vi "Get Drive List.vi"(7 "error in (no error)":errorcluster) -> (0 "error out":errorcluster, 3 "驱动器列表":string[](array[string]))   [LabVIEW 2012, in "API.lvlib"]
doc: "Uses an API call to retrieve a list of all available drives.\nThe output is an array of strings (one element for each drive letter)\nof the format \"c:\\\""
uses:
  API.lvlib
  kernel32.dll
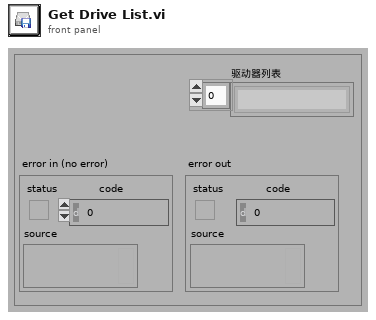
[diagram p1: front panel]
types:
  T1 = enum16{"big-endian, network order", "native, host order", "little-endian"}
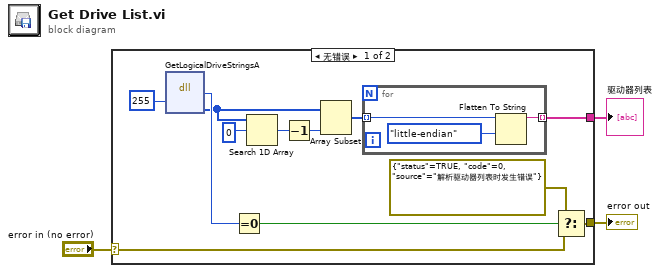
[diagram p0: block diagram]
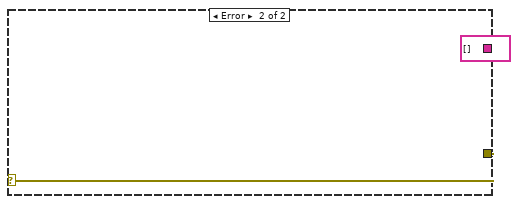
[diagram p2: hidden frame]
diagram:
  n1 = case shown="无错误" "error in (no error)" {
    selector: "error in (no error)" -> [w10 w19]
    tunnel: [w4 string[] []] -> w2
    tunnel: [w12 w19] -> w3
    frame No Error {
      n2 = dll-call lib="kernel32.dll" fn="GetLogicalDriveStringsA" ("GetLogiicalDriveStrings")("nBufferLength"=255) -> ("返回类型"=w14:u32, "lpBuffer"=w6:i32[])  [unwired: 4 in, 3 out]
      n3 = Equal To 0?(x=w14) -> (x = 0?=w11:bool)
      n4 = Search 1D Array(1D array=w6, element=0 ("元素")) -> (index of element=w8:i32)  [unwired: 1 in]
      n5 = Decrement(x=w8) -> (x-1=w7:i32)
      n6 = Array Subset(array=w6, length=w7) -> (w5:i32[])  [unwired: 1 in]
      n7 = for {
        tunnel: w5 -> [w17] mode=indexing
        tunnel: [w16] -> w4 mode=indexing
        n8 = Flatten To String(anything=w17, byte order (0:big-endian, network order)=T1."little-endian" ("字节顺序(0:big-endian, network order)")) -> (data string=w16:string)  [unwired: 2 in, 2 out]
      }
      n9 = Select(t=errorcluster {"status"=TRUE, "code"=0, "source"="解析驱动器列表时发生错误"} ("error in (no error)"), s=w11, f=w10) -> (s? t:f=w12:errorcluster)
    }
    frame Error {
    }
  }
  "error out" <- w3
  "驱动器列表" <- w2
